vi "Load Category.vi"(8 "error in (no error)":errorcluster, 10 "Category Base Path":path, 11 "Category in":refnum<class "Category.lvclass">) -> (0 "error out":errorcluster, 3 "Category out":refnum<class "Category.lvclass">)   [LabVIEW 2015, in "Category Library.lvlib" / "Category.lvclass"]
uses:
  Category.lvclass
  Category.lvclass/Category.ctl
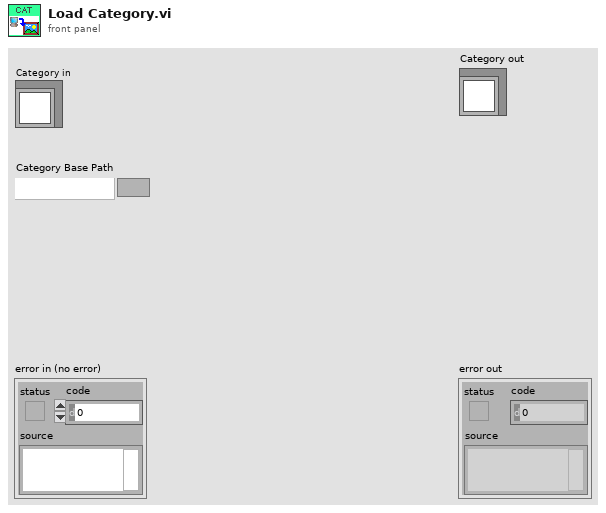
[diagram p1: front panel]
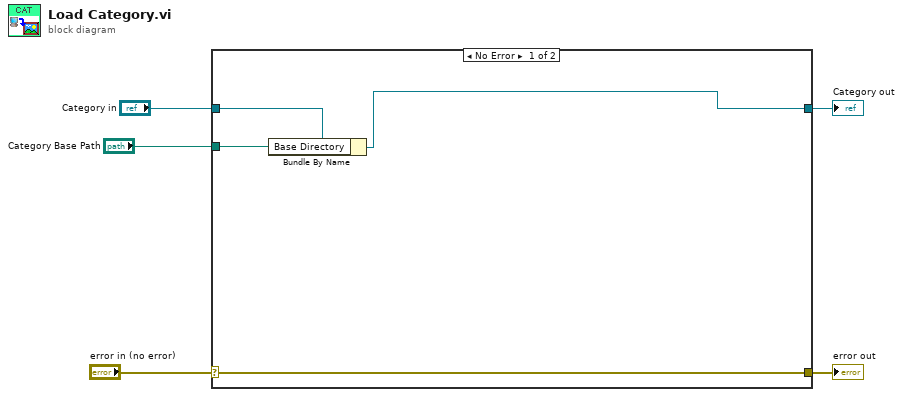
[diagram p0: block diagram]
diagram:
  n1 = case shown="No Error" "error in (no error)" {
    selector: "error in (no error)" -> [w9 w11]
    tunnel: [w9 w11] -> w4
    tunnel: [w6 w10] -> w2
    tunnel: "Category in" -> [w8 w10]
    tunnel: "Category Base Path" -> [w7 _]
    frame No Error {
      n2 = Bundle By Name(cluster=w8, "Base Directory"=w7) -> (w6:refnum<class "Category.lvclass">)
    }
    frame Error {
    }
  }
  "error out" <- w4
  "Category out" <- w2
